vi "C4Hdl_open.vi"() -> (4 "c4hdl out":refnum<k24>, 15 "error out":errorcluster)   [LabVIEW 2015, in "libC4HdlLV.lvlib"]
uses:
  libC4HdlLV.lvlib
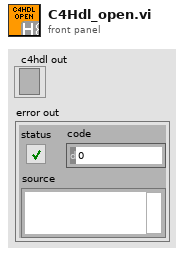
[diagram p1: front panel]
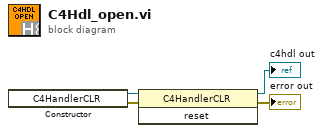
[diagram p0: block diagram]
diagram:
  n1 = constructor class="C4HandlerCLR"() -> (reference out=w4:refnum<k24>, error out=w3:errorcluster)  [unwired: 3 in, 1 out]
  n2 = invoke class="C4HandlerCLR" method="reset"(reference=w4, error in=w3) -> (reference out=→"c4hdl out":refnum<k24>, error out=→"error out":errorcluster)  [unwired: 1 in, 1 out]
